vi "Init ADCs.vi"(8 "Error IN":errorcluster, 11 "FPGA Ref":T1) -> (0 "error out":errorcluster, 2 "CFR":u64 format="%.0x", 3 "FPGA Ref Out":T1)   [LabVIEW 2013]
uses:
  Controls/FPGA_Reference.ctl
  <vilib>/Utility/error.llb/Error Cluster From Error Code.vi
  <vilib>/rvi/errors/niLvFpgaAdjustHostInterfaceError.vi
  <vilib>/rvi/interface/nirviReadWriteControl/nirviReadWriteControl.xnode
  FPGA/bitfiles/TI sbRIO PWM (FPGA) v1.0.lvbitx
  <userlib>/_NI SPI IP/FPGA/Controllers/Public/Transfer Settings.ctl
  NiFpgaLv.dll
  <userlib>/_NI SPI IP/FPGA/Controllers/DIO SPI FPGA.lvlib
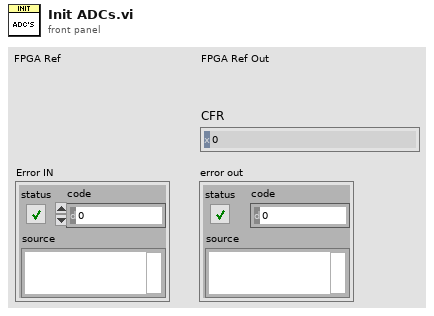
[diagram p1: front panel]
types:
  T1 = typedef "FPGA_Reference.ctl" = refnum<k20>
  T2 = cluster{"Divide Value":u8, "Transfer Length (bits)":u8, "CS Asserted Polarity":bool, "Clock Polarity (CPOL)":bool, "Clock Phase (CPHA)":bool, "Lengthen MISO Setup":bool, "Direction Change Bit":u8, "MOSI Starts as Output":bool, "Tristatable MOSI":bool}
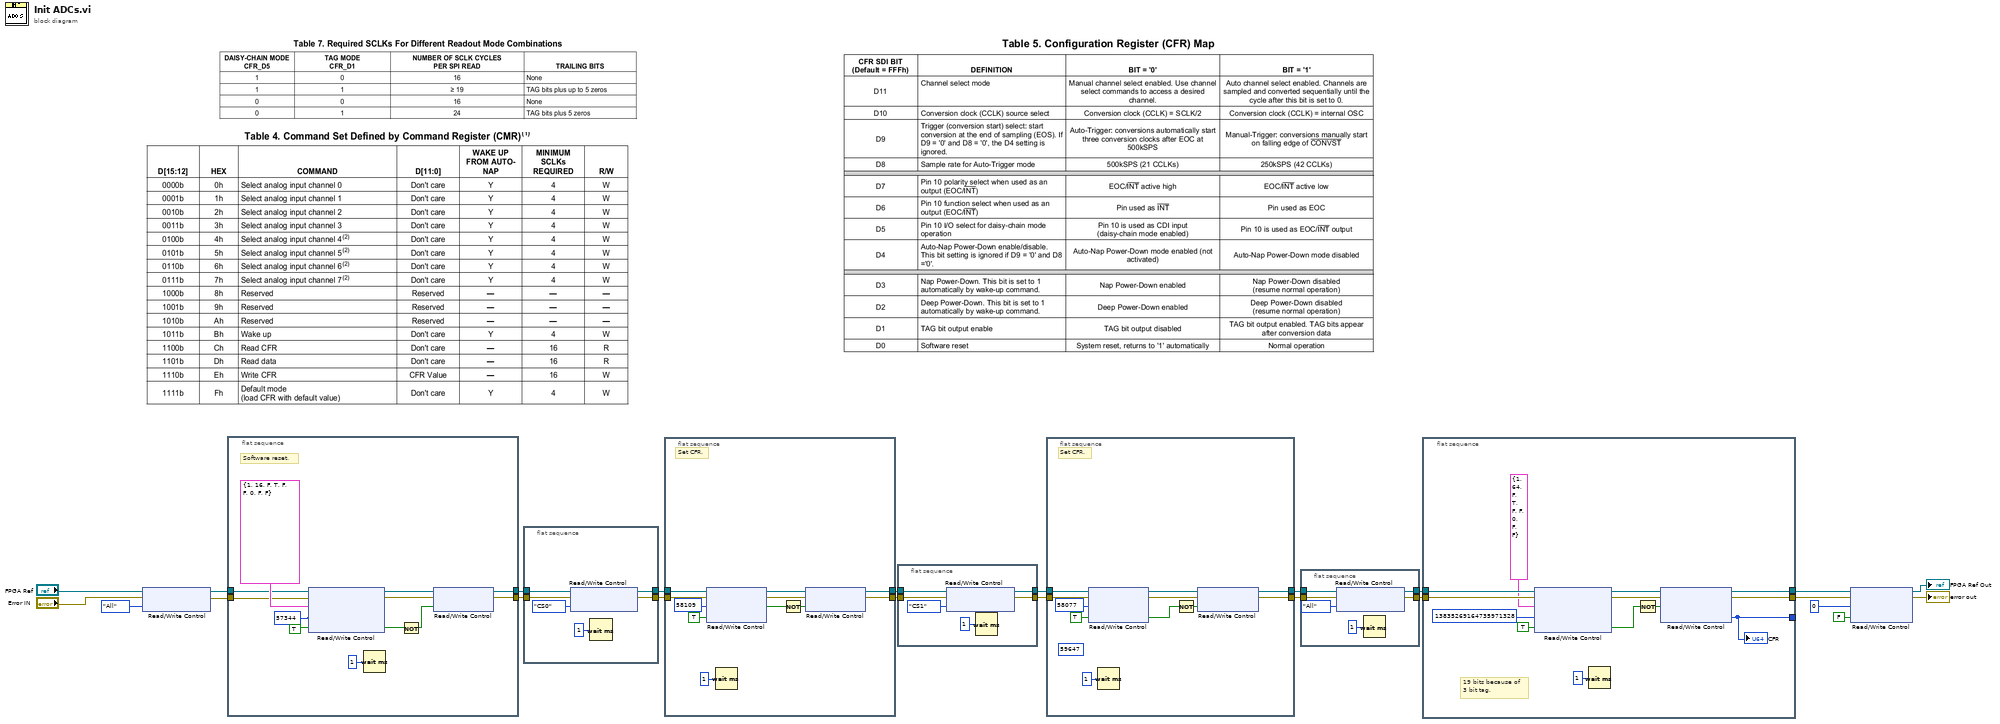
[diagram p0: block diagram]
diagram:
  n1 = xnode "Read/Write Control"("FPGA VI Reference In"="FPGA Ref", "error in"="Error IN", "ADC CS Mode"=enum16{"All", "CS0", "CS1"}."All" ("Mode")) -> ("FPGA VI Reference Out"=w4:T1, "error out"=w5:errorcluster)
  n2 = flat-sequence {
    tunnel: w4 -> [w33]
    tunnel: [w28] -> w7
    tunnel: w5 -> [w30]
    tunnel: [w25] -> w8
    frame #0 {
      w27 = TRUE ("Stop")
      # "Software reset."
      n3 = xnode "Read/Write Control"("FPGA VI Reference In"=w33, "error in"=w30, "ADC SPI Settings"=T2 {"Divide Value"=1, "Transfer Length (bits)"=16, "CS Asserted Polarity"=FALSE, "Clock Polarity (CPOL)"=TRUE, "Clock Phase (CPHA)"=FALSE, "Lengthen MISO Setup"=FALSE, "Direction Change Bit"=0, "MOSI Starts as Output"=FALSE, "Tristatable MOSI"=FALSE} ("Master Settings"), "ADC Data In"=u64 57344 ("data to write"), "ADC Trigger"=w27) -> ("FPGA VI Reference Out"=w29:T1, "error out"=w24:errorcluster)
      n4 = Wait (ms)(milliseconds to wait=u32 1) -> ()  [unwired: 1 out]
      n5 = Not(x=w27) -> (.not. x?=w26:bool)
      n6 = xnode "Read/Write Control"("FPGA VI Reference In"=w29, "error in"=w24, "ADC Trigger"=w26) -> ("FPGA VI Reference Out"=w28:T1, "error out"=w25:errorcluster)
    }
  }
  n7 = flat-sequence {
    tunnel: w7 -> [w40]
    tunnel: w8 -> [w39]
    tunnel: [w38] -> w9
    tunnel: [w37] -> w10
    frame #0 {
      n8 = xnode "Read/Write Control"("FPGA VI Reference In"=w40, "error in"=w39, "ADC CS Mode"=enum16{"All", "CS0", "CS1"}."CS0" ("Mode")) -> ("FPGA VI Reference Out"=w38:T1, "error out"=w37:errorcluster)
      n9 = Wait (ms)(milliseconds to wait=u32 1) -> ()  [unwired: 1 out]
    }
  }
  n10 = flat-sequence {
    tunnel: w9 -> [w50]
    tunnel: [w42] -> w13
    tunnel: w10 -> [w47]
    tunnel: [w41] -> w14
    frame #0 {
      w44 = TRUE ("Stop")
      # "Set CFR."
      n11 = xnode "Read/Write Control"("FPGA VI Reference In"=w50, "error in"=w47, "ADC Data In"=u64 58109 ("data to write"), "ADC Trigger"=w44) -> ("FPGA VI Reference Out"=w46:T1, "error out"=w45:errorcluster)
      n12 = Wait (ms)(milliseconds to wait=u32 1) -> ()  [unwired: 1 out]
      n13 = Not(x=w44) -> (.not. x?=w43:bool)
      n14 = xnode "Read/Write Control"("FPGA VI Reference In"=w46, "error in"=w45, "ADC Trigger"=w43) -> ("FPGA VI Reference Out"=w42:T1, "error out"=w41:errorcluster)
    }
  }
  n15 = flat-sequence {
    tunnel: [w55] -> w11
    tunnel: [w54] -> w12
    tunnel: w13 -> [w53]
    tunnel: w14 -> [w52]
    frame #0 {
      n16 = xnode "Read/Write Control"("FPGA VI Reference In"=w53, "error in"=w52, "ADC CS Mode"=enum16{"All", "CS0", "CS1"}."CS1" ("Mode")) -> ("FPGA VI Reference Out"=w54:T1, "error out"=w55:errorcluster)
      n17 = Wait (ms)(milliseconds to wait=u32 1) -> ()  [unwired: 1 out]
    }
  }
  n18 = flat-sequence {
    tunnel: w12 -> [w66]
    tunnel: w11 -> [w63]
    tunnel: [w58] -> w17
    tunnel: [w57] -> w15
    frame #0 {
      (unwired) u64 59647 ("data to write")
      w60 = TRUE ("Stop")
      # "Set CFR."
      n19 = xnode "Read/Write Control"("FPGA VI Reference In"=w66, "error in"=w63, "ADC Data In"=u64 58077 ("data to write"), "ADC Trigger"=w60) -> ("FPGA VI Reference Out"=w62:T1, "error out"=w61:errorcluster)
      n20 = Wait (ms)(milliseconds to wait=u32 1) -> ()  [unwired: 1 out]
      n21 = Not(x=w60) -> (.not. x?=w59:bool)
      n22 = xnode "Read/Write Control"("FPGA VI Reference In"=w62, "error in"=w61, "ADC Trigger"=w59) -> ("FPGA VI Reference Out"=w57:T1, "error out"=w58:errorcluster)
    }
  }
  n23 = flat-sequence {
    tunnel: w15 -> [w71]
    tunnel: [w70] -> w16
    tunnel: w17 -> [w69]
    tunnel: [w68] -> w18
    frame #0 {
      n24 = xnode "Read/Write Control"("FPGA VI Reference In"=w71, "error in"=w69, "ADC CS Mode"=enum16{"All", "CS0", "CS1"}."All" ("Mode")) -> ("FPGA VI Reference Out"=w68:T1, "error out"=w70:errorcluster)
      n25 = Wait (ms)(milliseconds to wait=u32 1) -> ()  [unwired: 1 out]
    }
  }
  n26 = flat-sequence {
    tunnel: w18 -> [w81]
    tunnel: [w82] -> w19
    tunnel: w16 -> [w79]
    tunnel: [w74] -> _
    tunnel: [w73] -> w22
    frame #0 {
      w75 = TRUE ("Stop")
      # "19 bits because of\n3 bit tag."
      n27 = xnode "Read/Write Control"("FPGA VI Reference In"=w81, "error in"=w79, "ADC SPI Settings"=T2 {"Divide Value"=1, "Transfer Length (bits)"=64, "CS Asserted Polarity"=FALSE, "Clock Polarity (CPOL)"=TRUE, "Clock Phase (CPHA)"=FALSE, "Lengthen MISO Setup"=FALSE, "Direction Change Bit"=0, "MOSI Starts as Output"=FALSE, "Tristatable MOSI"=FALSE} ("Master Settings 2"), "ADC Data In"=u64 13835269164735971328 ("data to write"), "ADC Trigger"=w75) -> ("FPGA VI Reference Out"=w84:T1, "error out"=w83:errorcluster)
      n28 = Wait (ms)(milliseconds to wait=u32 1) -> ()  [unwired: 1 out]
      n29 = Not(x=w75) -> (.not. x?=w76:bool)
      n30 = xnode "Read/Write Control"("FPGA VI Reference In"=w84, "error in"=w83, "ADC Trigger"=w76) -> ("FPGA VI Reference Out"=w82:T1, "error out"=w73:errorcluster, "ADC Read Data"=w74:u64)
      "CFR" <- w74
    }
  }
  n31 = xnode "Read/Write Control"("FPGA VI Reference In"=w19, "error in"=w22, "ADC Data In"=u64 0 ("nx-100 Data In"), "ADC Manual"=FALSE ("nx-100 Manual")) -> ("FPGA VI Reference Out"=→"FPGA Ref Out":T1, "error out"=→"error out":errorcluster)
